vi "Rcv1.vi"(8 "error in (no error)":errorcluster caption="entrée d'erreur (pas d'erreur)", 11 "fetch_rcv1":T2={"subset"="all", "download_if_missing"=TRUE, "random_state"=0, "shuffle"=TRUE, "Returns"="Data"} {"random_state" min=-1}) -> (0 "error out":errorcluster, 3 "Data":T1)   [LabVIEW 2020]
doc: "Reuters Corpus Volume I (RCV1) is an archive of over 800,000 manually categorized newswire stories made available by Reuters, Ltd. for research purposes. \n\nData Set Characteristics :\n - Classes : 103\n - Samples total : 804414\n - Dimensionality : 47236\n - Features : real, between 0 and 1\n\ndata : The feature matrix is a scipy CSR sparse matrix, with 804414 samples and 47236 features. Non-zero values contains cosine-normalized, log TF-IDF vectors. A nearly chronological split is proposed in 1: The first 23149 samples are the training set. The last 781265 samples are the testing set. This follows the official LYRL2004 chronological split. The array has 0.16% of non zero values.\n\ntarget: The target values are stored in a scipy CSR sparse matrix, with 804414 samples and 103 categories. Each sample has a value of 1 in its categories, and 0 in others. The array has 3.15% of non zero values.\n\nParameters :\n\n- subset : string, ‘train’, ‘test’, or ‘all’, default=’all’\nSelect the dataset to load: ‘train’ for the training set (23149 samples), ‘test’ for the test set (781265 samples), ‘all’ for both, with the training samples first if shuffle is False. This follows the official LYRL2004 chronological split.\n\n- download_if_missing : boolean, default=True\nIf False, raise a IOError if the data is not locally available instead of trying to download the data from the source site.\n\n- random_state : int, RandomState instance, default=None=-1\nDetermines random number generation for dataset shuffling. Pass an int for reproducible output across multiple function calls. See Glossary.\n\n- shuffle : bool, default=False\nWhether to shuffle dataset.\n\n\nReturns :\n\n- data : scipy csr array, dtype np.float64, shape (804414, 47236)\nThe array has 0.16% of non zero values.\n\n- target : scipy csr array, dtype np.uint8, shape (804414, 103)\nEach sample has a value of 1 in its categories, and 0 in others. The array has 3.15% of non zero values."
uses:
  Rcv1.lvclass
panel:
  out "Rcv1.lvclass":refnum<class "Rcv1.lvclass">
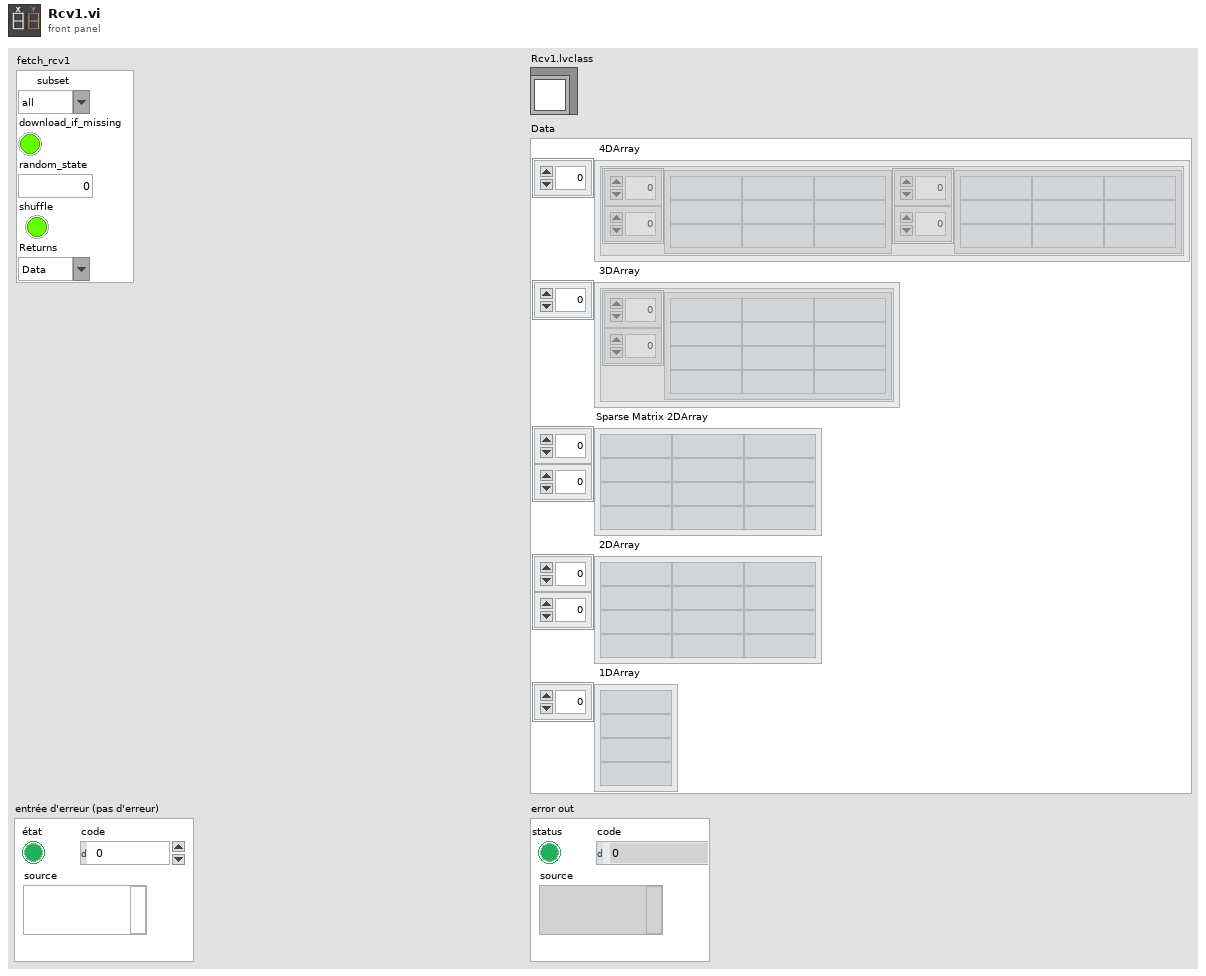
[diagram p1: front panel]
types:
  T1 = cluster{" 4DArray":cluster{"1":string[][], "2":string[][]}[], " 3DArray":cluster{"Tableau":string[][]}[], "Sparse Matrix 2DArray":string[][], " 2DArray":string[][], " 1DArray":string[]}
  T2 = cluster{"subset":string, "download_if_missing":bool, "random_state":i32, "shuffle":bool, "Returns":string}
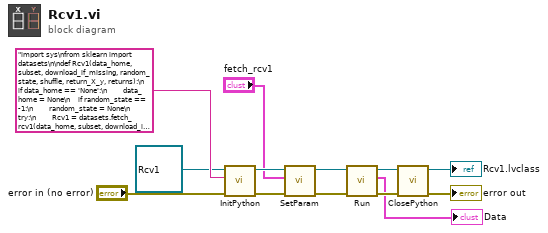
[diagram p0: block diagram]
diagram:
  n1 = call-dynamic "InitPython.vi"("error in (no error)"="error in (no error)", "Python Instruction"="import sys\nfrom sklearn import datasets\n\ndef Rcv1(data_home, subset, download_if_missing, random_state, shuffle, return_X_y, returns):\n    if data_home == 'None':\n        data_home = None\n    if random_state == -1:\n        random_state = None\n    try:\n        Rcv1 = datasets.fetch_rcv1(data_home, subset, download_if_missing, random_state, shuffle, return_X_y)\n        if returns == 'Data': \n            data = Rcv1['data']\n            Mat = data.tocoo()\n            return str(list(zip(Mat.row, Mat.col, Mat.data)))\n        else :\n            data = Rcv1['target']\n            Mat = data.tocoo()\n            return str(list(zip(Mat.row, Mat.col, Mat.data)))\n    except:\n        erreur = sys.exc_info()\n        typerr = u\"%s\" % (erreur[0])\n        typerr = typerr[typerr.find(\"'\")+1:typerr.rfind(\"'\")]\n        msgerr = u\"%s\" % (erreur[1])\n        message = str('/!\\\\ {0} : {1}'. format(typerr,msgerr))\n        return message", "Scikit-learn en entrée"=refnum<class "Rcv1.lvclass"> refnum ("Rcv1.lvclass")) -> ("error out"=w9:errorcluster, "Scikit-learn en sortie"=w10:refnum<class "Rcv1.lvclass">)  [unwired: 7 in]
  n2 = call-dynamic "SetParam.vi"("error in (no error)"=w9, "fetch_rcv1"="fetch_rcv1", "Rcv1.lvclass"=w10) -> ("error out"=w6:errorcluster, "Rcv1.lvclass"=w7:refnum<class "Rcv1.lvclass">)  [unwired: 7 in]
  n3 = call-dynamic "Run.vi"("error in (no error)"=w6, "Rcv1.lvclass"=w7) -> ("error out"=w4:errorcluster, "Data"=→"Data":T1, "Rcv1.lvclass"=w5:refnum<class "Rcv1.lvclass">)  [unwired: 7 in]
  n4 = call-dynamic "ClosePython.vi"("error in (no error)"=w4, "Scikit-learn en entrée"=w5) -> ("error out"=→"error out":errorcluster, "Scikit-learn en sortie"=→"Rcv1.lvclass":refnum<class "Rcv1.lvclass">)  [unwired: 8 in]
